vi "Cross Product.vi"(10 "B Vector":dbl[](array[numeric]), 11 "A Vector":dbl[](array[numeric])) -> (0 "error":i32, 3 "Cross Product":dbl[](array[numeric]))   [LabVIEW 2020, in "NI_AALPro.lvlib"]
doc: "Calculates the cross product of <B>A Vector</B> and <B>B Vector</B>."
uses:
  <vilib>/Analysis/NI_AALPro.lvlib
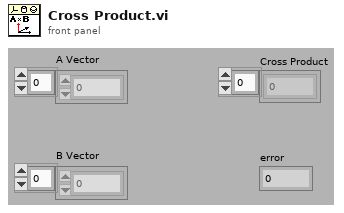
[diagram p1: front panel]
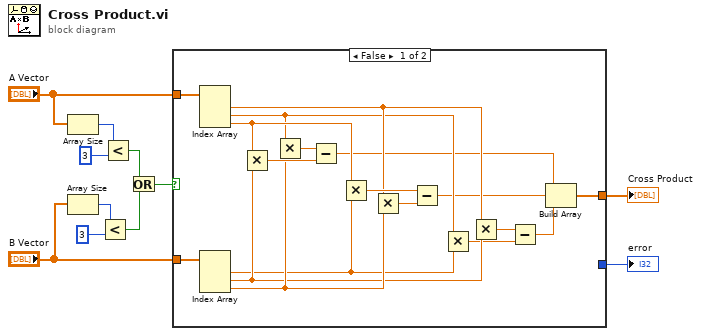
[diagram p0: block diagram]
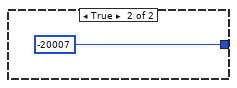
[diagram p2: hidden frame]
diagram:
  n1 = Array Size(array="A Vector") -> (size(s)=w8:i32)
  n2 = Array Size(array="B Vector") -> (size(s)=w6:i32)
  n3 = Less?(x=w6, y=3) -> (x < y?=w3:bool)
  n4 = Less?(x=w8, y=3) -> (x < y?=w4:bool)
  n5 = Or(x=w4, y=w3) -> (x .or. y?=w2:bool)
  n6 = case shown="False" w2 {
    tunnel: [w14 _] -> w11
    tunnel: "A Vector" -> [w13 _]
    tunnel: "B Vector" -> [w12 _]
    tunnel: [_ -20007] -> w1
    frame False {
      n7 = Index Array(array=w13) -> (element #1=w23:dbl, element #2=w21:dbl, element #3=w26:dbl)  [unwired: 3 in]
      n8 = Index Array(array=w12) -> (element #1=w20:dbl, element #2=w22:dbl, element #3=w27:dbl)  [unwired: 3 in]
      n9 = Multiply(x=w26, y=w22) -> (x*y=w28:dbl)
      n10 = Multiply(x=w21, y=w27) -> (x*y=w29:dbl)
      n11 = Subtract(x=w29, y=w28) -> (x-y=w16:dbl)
      n12 = Multiply(x=w26, y=w20) -> (x*y=w25:dbl)
      n13 = Multiply(x=w23, y=w27) -> (x*y=w24:dbl)
      n14 = Subtract(x=w25, y=w24) -> (x-y=w15:dbl)
      n15 = Multiply(x=w21, y=w20) -> (x*y=w18:dbl)
      n16 = Multiply(x=w23, y=w22) -> (x*y=w19:dbl)
      n17 = Subtract(x=w19, y=w18) -> (x-y=w17:dbl)
      n18 = Build Array(w16, w15, w17) -> (w14:dbl[])
    }
    frame True {
    }
  }
  "Cross Product" <- w11
  "error" <- w1
